vi "ReadWriteHWIO.vi"(0 "HWIO Configuration List 3":string[][](table), 3 "error in":errorcluster, 4 "Enum":enum16{"default", "Write", "Read"}(ring)) -> (7 "HWIO Configuration List 2":string[][](array[string]), 10 "error out":errorcluster)   [LabVIEW 2015]
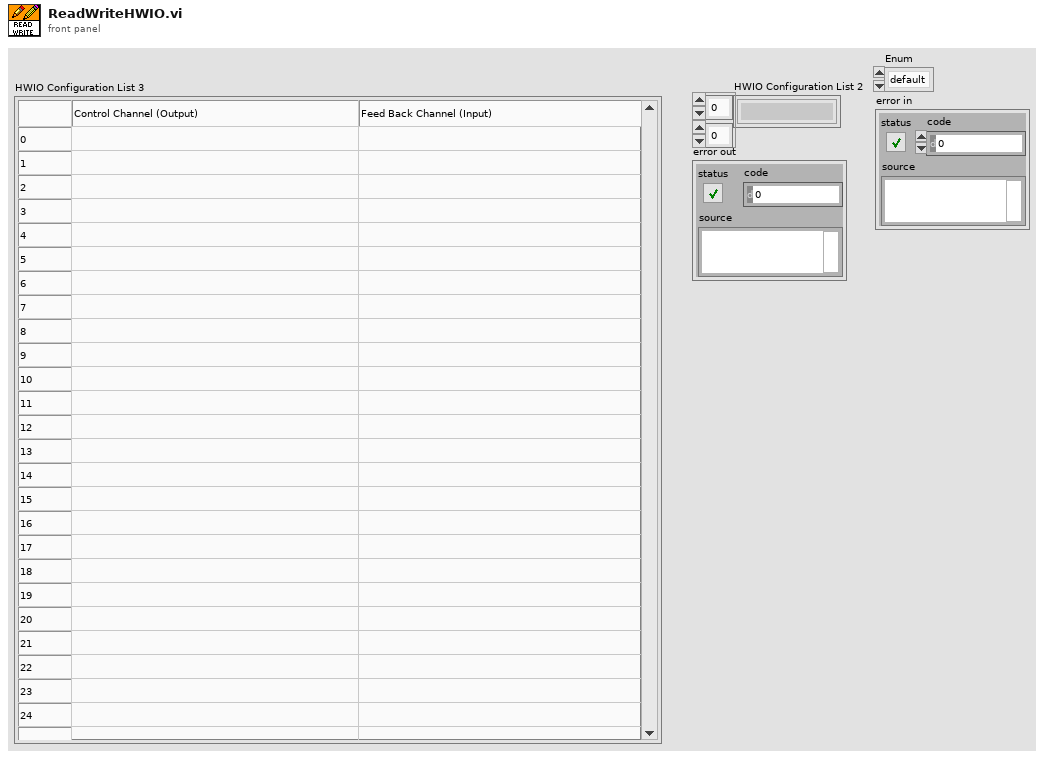
[diagram p1: front panel]
types:
  T1 = enum16{"open", "replace", "create", "open or create", "replace or create", "replace or create with confirmation"}
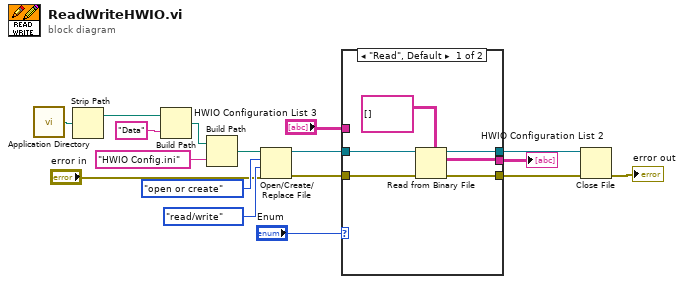
[diagram p0: block diagram]
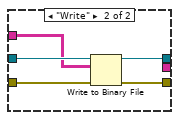
[diagram p2: hidden frame]
diagram:
  n1 = call <vilib>:"Application Directory.vi"() -> ("Application Directory"=w3:path)
  n2 = Strip Path(path=w3) -> (stripped path=w4:path)  [unwired: 1 out]
  n3 = Build Path(base path=w4, name or relative path="Data") -> (appended path=w6:path)
  n4 = Build Path(base path=w6, name or relative path="HWIO Config.ini") -> (appended path=w7:path)
  n5 = Open/Create/Replace File(file path (use dialog)=w7, error in="error in", operation (0:open)=T1."open or create", access (0:read/write)=enum16{"read/write", "read-only", "write-only"}."read/write") -> (refnum out=w11:refnum<file>, error out=w12:errorcluster)  [unwired: 2 in, 1 out]
  n6 = case shown="\"Read\", Default" "Enum" {
    tunnel: w11 -> [w23 w28]
    tunnel: w12 -> [w22 w27]
    tunnel: "HWIO Configuration List 3" -> [_ w26]
    tunnel: [w20 w25] -> w14
    tunnel: [w19 w24] -> w15
    tunnel: [w18 _] -> w13
    frame "Read", Default {
      n7 = Read from Binary File(5:string[][] [] ("HWIO Configuration List"), 8:w22, 11:w23) -> (0:w19:errorcluster, 2:w18:string[][], 3:w20:refnum<file>)  [unwired: 3 in, 1 out]
    }
    frame "Write" {
      n8 = Write to Binary File(file (use dialog)=w28, data=w26, error in=w27) -> (refnum out=w25:refnum<file>, error out=w24:errorcluster)  [unwired: 3 in, 1 out]
    }
  }
  "HWIO Configuration List 2" <- w13
  n9 = Close File(refnum=w14, error in=w15) -> (error out=→"error out":errorcluster)  [unwired: 1 out]
